vi "AlliGator Decay Window.vi"() -> ()   [LabVIEW 2021, in "AlliGator Local Decay Window.lvlib"]
doc: "Local Decay Window UI.\nThis window displays the decay (and when available, IRF, fit and residuals) at the selected ROI."
uses:
  AlliGator Local Decay Window.lvlib
  AlliGator Variables List.ctl
  AlliGator Local Decay Graph Window Event Refnum.ctl
  AlliGator Local Decay Fit Results.ctl
  AlliGator Image Profile Plot Data.ctl
  Graphs/XY Graph/XY Plot Data.ctl
  Graphs/XY Graph/XY Graph Refnum.ctl
  Graphs/XY Graph/XY Graph Event.ctl
  <vilib>/Utility/miscctls.llb/LVPoint32TypeDef.ctl
  Variant/Variant to Data/Variant to Boolean.vi
  Graphs/XY Graph/XY Graph Add-Ons.lvlib
  AlliGator Globals, Variables & Constants.lvlib
  AlliGator Image Profile Window.lvlib
  Notebook/Notebook.lvlib
  Rich Text Box/Rich Text Box.lvlib
  AlliGator Settings.lvlib
  Error/Error.lvlib
  Variant/Variant to Data/Variant to Data.lvlib
panel:
  out "Local Decay Graph TipStrip":string
  out "Local Decay Graph":cluster{"X Array":dbl[], "Y Array":dbl[]}[](graph)
  out "Expand top panel to increase Graph size/Expand lower panel to see fit results":string
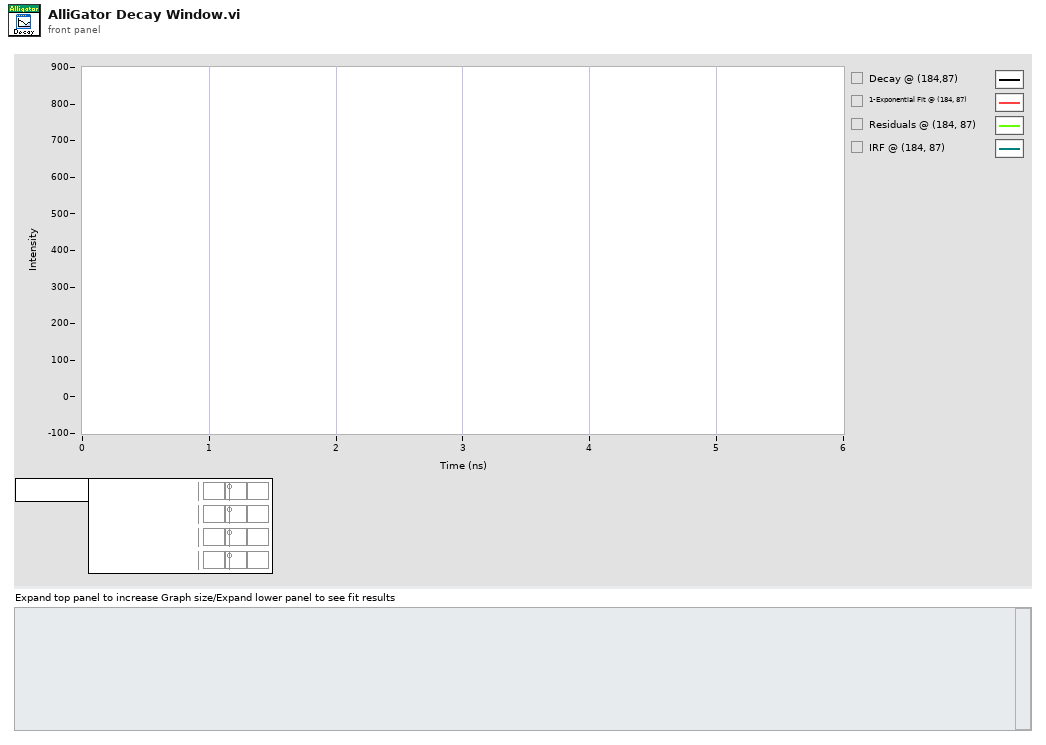
[diagram p1: front panel]
types:
  T1 = cluster{"Local Decay TipStrip Event":refnum<event-registration>, "Local Decay Window Event":refnum<event-registration>}
  T2 = typedef "AlliGator Local Decay Window.lvlib/AlliGator Local Decay Graph Window Event Refnum.ctl" = refnum<user-event>
  T3 = typedef "AlliGator Globals, Variables & Constants.lvlib/AlliGator Variables List.ctl" = enum16{"---- GUI ----", "Initialization Status", "State Indicators Refnum", "Original AlliGator Menu Items", "Current Action Loop State", "Script in progress", "Playback", "Loop Playback", "Search ROI Used", "Search ROI", "Decay Graph Max Legend Size", "Intensity Graph Max Legend Size", "Decay Statistics Graph Max Legend Size", "Phasor Graph Max Legend Size", "Phasor Ratio Graph Max Legend Size", "Lifetime Graph Max Legend Size", "---- Files ----", "Export Dataset Frames as Individual Files", "Show Batch Export Help Balloons", "Frames in Dataset", "ptu File Frame Start Indices", "Current Frame in Dataset", "Current Frame Timestamp", "------ Python Plugins ------", "Python Plugins Information", "Python Session", "Valid Python Session?", "---- Source Image ----", "Dataset Loaded", "Dataset Metadata", "Dataset Channel", "Dataset Data Description", "Background Dataset Metadata", "Background Dataset Channel", "Background Dataset Data Description", "Background File Subtraction", "Background File Path", "Background File Pile-up Correction", "Background File Pixel Well Capacity", "Background File Scaling Factor", "Source Image ROIs", "Current Source Image ROI", "Source Image ROI Event Refnum", "X_Source Image Display Range", "X_Source Image Palette Information", "Source Image Palette List", "Source Image Scale", "Current Dataset Load Settings", "Source Image:ROI Overlay Color", "---- Image Profile Window ----", "Image Profile:Overlay ROI in Source Image", "Image Profile Window Event Refnum", "Image Profile:IntensityType", "Image Profile:Intensity Average Type", "Image Profile:Intensity-weighted SDV", "Image Profile:Box Profile Type", "Image Profile Window Open", "Image Profile:Plotted Fit Parameter", "X_Type of Displayed Image", "X_Time Gate Slider", "Dataset Path", "Source Image Overlay to Erase", "Is Displayed Image Accumulated", "White Light Image Modified", "Mask Image Modified", "Macrotime Gate Separation", "------ Phasor Graph -------", "Phasor Graph:Show Line", "---- Phasor Plot ---", "Phasor Plot Parameters Changed", "FLI Dataset Modified since last Phasor Plot Calculation", "Phasor Harmonics Data", "Selected Phasor Harmonics", "Phasor Harmonic Manager Event Refnum", "Phasor Plot ROIs", "Current Phasor Plot ROI", "Phasor Plot ROI Event Refnum", "Phasor Plot Image Reference Points", "Phasor Plot Computed", "Phasor Plot Palette Information", "Phasor Plot Palette List", "Phasor Ratio Palette Information", "Phasor Ratio Palette List", "Phasor Image Scale", "Phasor Plot Image Overlay to Erase", "Phasor Plot Image Elements to Update", "Current Phasor Plot Calculation Parameters", "Current Phasor Calibration Options", "Reset Cumulated Phasor Plot", "Phasor Ratio Reference 1", "Phasor Ratio Lifetime Reference 1", "Phasor Ratio Reference 1 Frequency", "Phasor Ratio Reference 2", "Phasor Ratio Lifetime Reference 2", "Phasor Ratio Reference 2 Frequency", "---- Decay Analysis ----", "Number of Selected Decays to Fit", "LS Fit Results", "LAR Fit Results", "BS Fit Results", "Last Decay Max - Min", "Best Fit Parameters", "Best Fit Parameter Names", "Actual Size X", "Actual Size Y", "Binning X", "Binning Y", "Actual # Gates", "Dataset Number", "Gates to...", "Gates Skipped", "Gates to keep", "Gate Step", "Gate Separation", "Reversed Gates", "Pile-up Correction", "Pixel Well Capacity", "Background Subtracted", "Background Subtraction Method", "Background Definition Range", "Background File (deprecated)", "Number of Dataset Accumulated", "Array of Accumulated Dataset Paths", "Do Averaged Datasets", "Destination File Path", "Process Plot Target", "Use 1/D as Phasor Frequency", "---- Decay Fit Parameter Map -----", "Decay Fit Parameter Map Palette Information", "Decay Fit Parameter Map Palette List", "Local Decay Graph Window Event Refnum", "------- Local Decay Window ---------", "Use normalized IRF for convolution", "----- Miscellaneous ----", "Skippable Dialog Windows Status"}
  T4 = typedef "XY Graph Add-Ons.lvlib/XY Graph Refnum.ctl" = refnum<vi>
  T5 = typedef "XY Graph Add-Ons.lvlib/XY Graph Event.ctl" = cluster{"Item Tag":string, "XY Graph Refnum":refnum<vi>, "Coords":T6, "Item Path":string}
  T6 = typedef "LVPoint32TypeDef.ctl" = cluster{"Horizontal":i32, "Vertical":i32}
  T7 = typedef "Rich Text Box.lvlib/Text Formatting.ctl" = cluster{"Font":string, "Text Color":T8, "Text Background Color":T8, "Text Style":enum16{"Regular", "Bold", "Italic", "Underline", "Strikeout"}, "Font Size (Points)":dbl, "Text Alignment":i32}
  T8 = typedef "Rich Text Box.lvlib/Text Colors.ctl" = enum16{"Unchanged", "Black", "Blue", "Brown", "Gray", "Green", "Orange", "Pink", "Red", "White"}
  T9 = typedef "AlliGator Image Profile Window.lvlib/AlliGator Image Profile Plot Data.ctl" = cluster{"Plot Name":string, "Plot":T10}
  T10 = typedef "XY Graph Add-Ons.lvlib/XY Plot Data.ctl" = cluster{"X Array":dbl[], "Y Array":dbl[]}
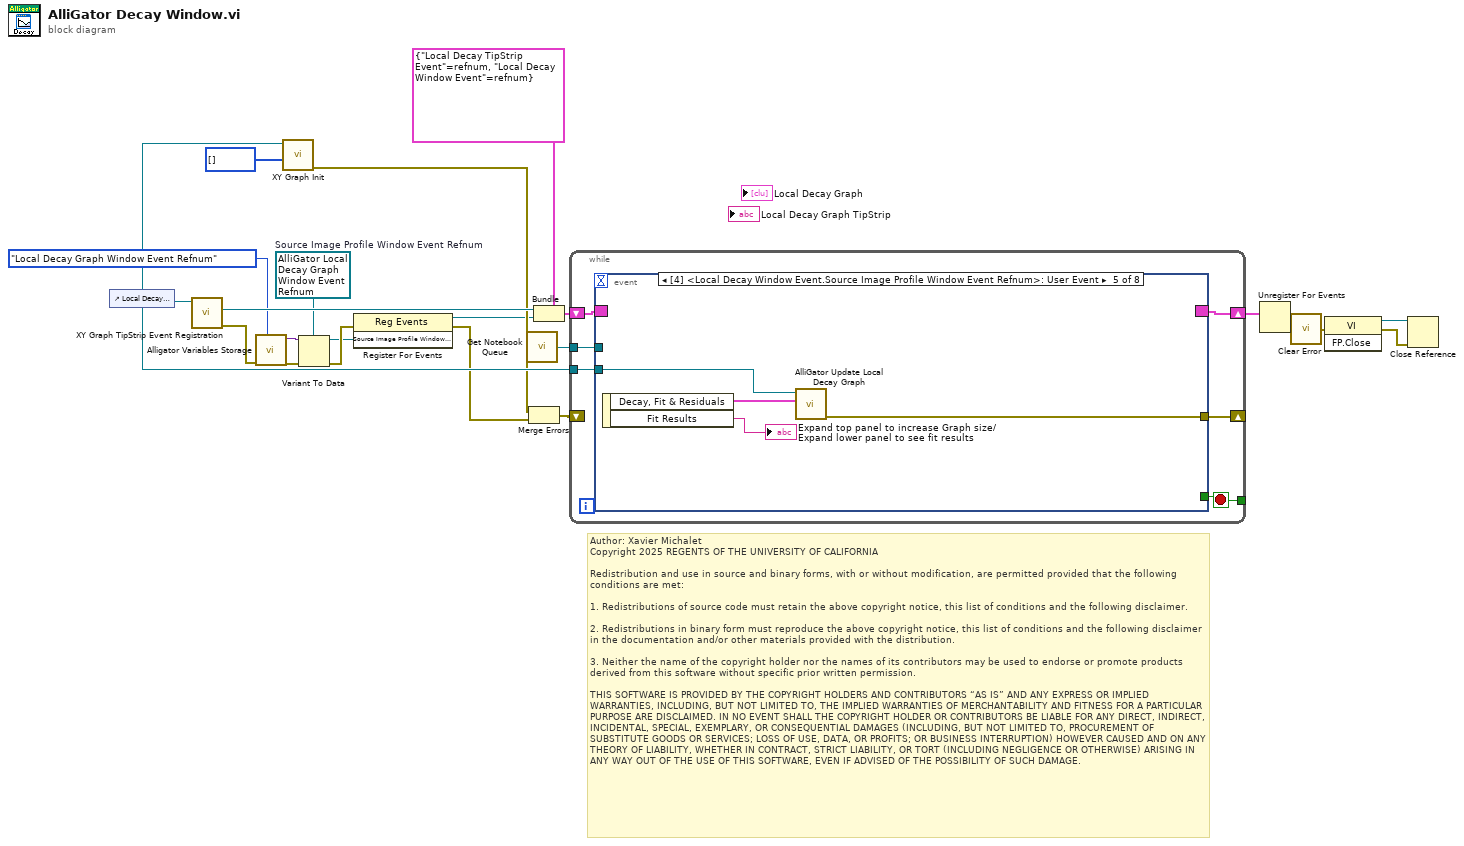
[diagram p0: block diagram]
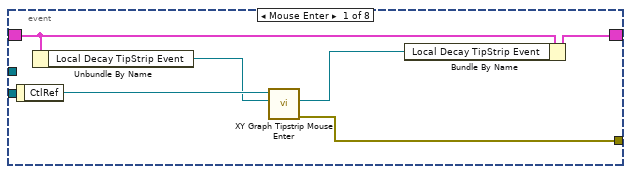
[diagram p2: hidden frame]
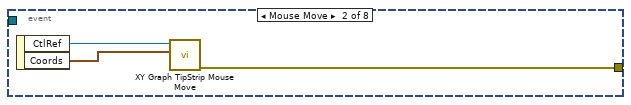
[diagram p3: hidden frame]
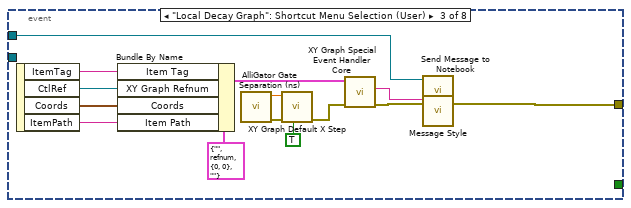
[diagram p4: hidden frame]
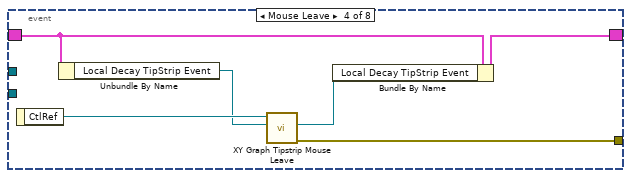
[diagram p5: hidden frame]
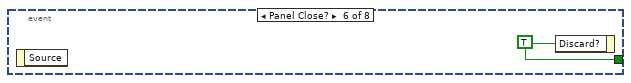
[diagram p6: hidden frame]
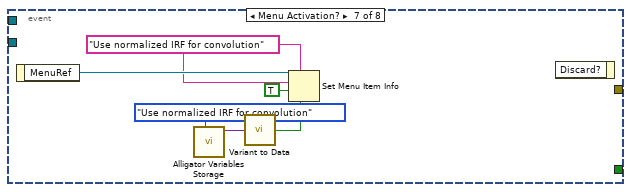
[diagram p7: hidden frame]
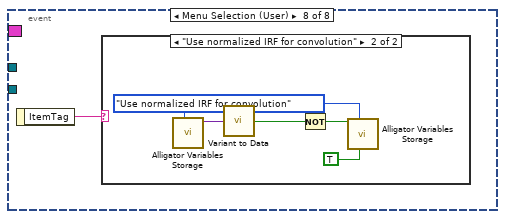
[diagram p8: hidden frame]
diagram:
  w15 = T2 refnum  # Source Image Profile Window Event Refnum
  # "Author: Xavier Michalet\nCopyright 2025 REGENTS OF THE UNIVERSITY OF CALIFORNIA\n\nRedistribution and use in source and binary forms, with or without modification, are permitted provided that the following conditions are met:\n\n1. Redistributions of source code must retain the above copyright notice, this list of conditions and the following disclaimer.\n\n2. Redistributions in binary form must reproduce the above copyright notice, this list of conditions and the following disclaimer in the documentation and/or other materials provided with the distribution.\n\n3. Neither the name of the copyright holder nor the names of its contributors may be used to endorse or promote products derived from this software without specific prior written permission.\n\nTHIS SOFTWARE IS PROVIDED BY THE COPYRIGHT HOLDERS AND CONTRIBUTORS “AS IS” AND ANY EXPRESS OR IMPLIED WARRANTIES, INCLUDING, BUT NOT LIMITED TO, THE IMPLIED WARRANTIES OF MERCHANTABILITY AND FITNESS FOR A PARTICULAR PURPOSE ARE DISCLAIMED. IN NO EVENT SHALL THE COPYRIGHT HOLDER OR CONTRIBUTORS BE LIABLE FOR ANY DIRECT, INDIRECT, INCIDENTAL, SPECIAL, EXEMPLARY, OR CONSEQUENTIAL DAMAGES (INCLUDING, BUT NOT LIMITED TO, PROCUREMENT OF SUBSTITUTE GOODS OR SERVICES; LOSS OF USE, DATA, OR PROFITS; OR BUSINESS INTERRUPTION) HOWEVER CAUSED AND ON ANY THEORY OF LIABILITY, WHETHER IN CONTRACT, STRICT LIABILITY, OR TORT (INCLUDING NEGLIGENCE OR OTHERWISE) ARISING IN ANY WAY OUT OF THE USE OF THIS SOFTWARE, EVEN IF ADVISED OF THE POSSIBILITY OF SUCH DAMAGE."
  n1 = control-ref of="Local Decay Graph"() -> (w19:refnum<vi>)
  n2 = call "XY Graph TipStrip Event Registration.vi"("XY Graph Refnum"=w19) -> ("error out"=w9:errorcluster, "Event Registration Refnum"=w21:refnum<event-registration>, "XY Graph Refnum"=w20:T4)  [unwired: 8 in]
  n3 = call "Alligator Variables Storage.vi"("AlliGator Variable"=AlliGator_Variables_List."Local Decay Graph Window Event Refnum" ("Alligator Variable"), "Error In"=w9) -> ("Error Out"=w16:errorcluster, "Data out"=w17:variant)  [unwired: 7 in, 1 out]
  n4 = call "XY Graph Init.vi"("Plots to Skip (none)"=i32[] [], "XYGraph in"=w20) -> ("Error Out"=w8:errorcluster)  [unwired: 9 in]
  n5 = Variant To Data(error in=w16, type=w15, Variant=w17) -> (data=w6:T2, error out=w14:errorcluster)
  n6 = register-events(error in=w14, w6) -> (reference out=w7:refnum<event-registration>, error out=w5:errorcluster)  [unwired: 1 in]
  n7 = call "Get Notebook Queue.vi"() -> ("Notebook Queue"=w11:refnum<queue>)  [unwired: 9 in]
  n8 = Merge Errors(w8, w5) -> (w10:errorcluster)
  n9 = Bundle(cluster=T1 {"Local Decay TipStrip Event"=refnum, "Local Decay Window Event"=refnum}, "Local Decay TipStrip Event"=w21, "Local Decay Window Event"=w7) -> (w12:T1)
  n10 = while {
    shift-right: [w28] -> w22
    shift-left: w12 -> [w29]
    tunnel: w19 -> [w27]
    tunnel: w11 -> [w26]
    shift-right: [w25] -> _
    shift-left: w10 -> [_]
    tunnel: [w24] -> _
    stop <- w24 stop-if-true
    n11 = event shown="[4] <Local Decay Window Event.Source Image Profile Window Event Refnum>: User Event" {
      selector: w29 -> [w33 _ _ w56 _ _ _ _]
      dyn-events: [w35 _ _ w55 _ _ _ _] -> w28
      timeout: _ -> [_ _ _ _ _ _ _ _]
      tunnel: [_ _ _ _ _ w64 _ _] -> w24
      tunnel: w27 -> [_ _ _ _ w63 _ _ _]
      tunnel: w26 -> [_ _ w51 _ _ _ _ _]
      tunnel: [w30 w36 w49 w54 w62 _ _ _] -> w25
      event Mouse Enter {
        n12 = event-data() -> ("CtlRef"=w34:refnum<vi>)  [unwired: 1 in]
        n13 = Unbundle By Name(w33) -> ("Local Decay TipStrip Event"=w32:refnum<event-registration>)
        n14 = call "XY Graph Tipstrip Mouse Enter.vi"("Event Registration Refnum"=w32, "XY Graph Refnum"=w34) -> ("Error Out"=w30:errorcluster, "Event Registration Refnum"=w31:refnum<event-registration>)  [unwired: 8 in]
        n15 = Bundle By Name(cluster=w33, "Local Decay TipStrip Event"=w31) -> (w35:T1)
      }
      event Mouse Move {
        n16 = event-data() -> ("CtlRef"=w38:refnum<vi>, "Coords"=w37:T6)  [unwired: 1 in]
        n17 = call "XY Graph TipStrip Mouse Move.vi"("Coords"=w37, "XY Graph Refnum"=w38) -> ("Error Out"=w36:errorcluster)  [unwired: 7 in, 2 out]
      }
      event "Local Decay Graph": Shortcut Menu Selection (User) {
        n18 = event-data() -> ("ItemTag"=w48:string, "CtlRef"=w47:refnum<vi>, "Coords"=w46:T6, "ItemPath"=w45:string)  [unwired: 1 in]
        n19 = Bundle By Name(cluster=T5 {"Item Tag"="", "XY Graph Refnum"=refnum, "Coords"={"Horizontal"=0, "Vertical"=0}, "Item Path"=""} ("XY Graph Event"), "Item Tag"=w48, "XY Graph Refnum"=w47, "Coords"=w46, "Item Path"=w45) -> (w43:T5)
        n20 = call "AlliGator Gate Separation (ns).vi"() -> ("error out"=w42:errorcluster, "Gate Separation (ns)"=w40:dbl)  [unwired: 10 in]
        n21 = call "XY Graph Default X Step.vi"("Get (F)/Set"=TRUE, "Error In"=w42, "Default X Step"=w40) -> ("Error Out"=w41:errorcluster)  [unwired: 7 in, 1 out]
        n22 = call "XY Graph Special Event Handler Core.vi"("error in (no error)"=w41, "XY Graph Event"=w43) -> ("error out"=w53:errorcluster, "Message"=w52:string)  [unwired: 5 in, 3 out]
        n23 = call "Message Style.vi"() -> ("Message Formatting"=w50:T7)
        n24 = call "Send Message to Notebook.vi"("Text Formatting"=w50, "Error In"=w53, "Message"=w52, "Notebook Queue"=w51) -> ("Error Out"=w49:errorcluster)  [unwired: 4 in, 1 out]
      }
      event Mouse Leave {
        n25 = event-data() -> ("CtlRef"=w59:refnum<vi>)  [unwired: 1 in]
        n26 = Unbundle By Name(w56) -> ("Local Decay TipStrip Event"=w58:refnum<event-registration>)
        n27 = call "XY Graph Tipstrip Mouse Leave.vi"("Event Registration Refnum"=w58, "XY Graph Refnum"=w59) -> ("Error Out"=w54:errorcluster, "Event Registration Refnum"=w57:refnum<event-registration>)  [unwired: 8 in]
        n28 = Bundle By Name(cluster=w56, "Local Decay TipStrip Event"=w57) -> (w55:T1)
      }
      event User Event {
        n29 = event-data() -> ("Decay, Fit & Residuals"=w61:T9[], "Fit Results"=→"Expand top panel to increase Graph size/Expand lower panel to see fit results":string)  [unwired: 1 in]
        n30 = call "AlliGator Update Local Decay Graph.vi"("Profile Window Data"=w61, "XY Graph Refnum"=w63) -> ("Error Out"=w62:errorcluster)  [unwired: 9 in]
      }
      event Panel Close? {
        w64 = TRUE ("Discard?")
        n31 = event-data() -> ()  [unwired: 1 in, 1 out]
        n32 = event-data("Discard?"=w64) -> ()  [unwired: 1 in, 1 out]
      }
      event Menu Activation? {
        w66 = "Use normalized IRF for convolution" ("item tag")
        n33 = event-data() -> ("MenuRef"=w70:refnum<k9>)  [unwired: 1 in]
        n34 = call "Alligator Variables Storage.vi"("AlliGator Variable"=AlliGator_Variables_List."Use normalized IRF for convolution") -> ("Data out"=w68:variant)  [unwired: 8 in, 2 out]
        n35 = call-poly "Variant to Data.vi"("Variant"=w68) -> ("Value"=w67:bool)  [unwired: 8 in]
        n36 = Set Menu Item Info(6:w67, 7:w66, 9:TRUE ("enabled"), 10:w66, 11:w70) -> ()  [unwired: 2 in, 2 out]
        n37 = event-data() -> ()  [unwired: 2 in, 1 out]
      }
      event Menu Selection (User) {
        n38 = event-data() -> ("ItemTag"=w71:string)  [unwired: 1 in]
        n39 = case shown="\"Use normalized IRF for convolution\"" w71 {
          frame "", Default {
          }
          frame "Use normalized IRF for convolution" {
            w72 = AlliGator_Variables_List."Use normalized IRF for convolution" ("AlliGator Variable")
            n40 = call "Alligator Variables Storage.vi"("AlliGator Variable"=w72) -> ("Data out"=w76:variant)  [unwired: 8 in, 2 out]
            n41 = call-poly "Variant to Data.vi"("Variant"=w76) -> ("Value"=w75:bool)  [unwired: 8 in]
            n42 = Not(x=w75) -> (.not. x?=w74:bool)
            n43 = call "Alligator Variables Storage.vi"("Get(F)/Set"=TRUE, "AlliGator Variable"=w72, "Data in"=w74) -> ()  [unwired: 6 in, 3 out]
          }
        }
      }
    }
  }
  n44 = Unregister For Events(event registration refnum=w22) -> (error out=w4:errorcluster)  [unwired: 1 in]
  n45 = call "Clear Error.vi"("Error In"=w4) -> ("no Error Out"=w1:errorcluster)  [unwired: 8 in]
  n46 = invoke class="VI" method="FP.Close"(error in=w1) -> (reference out=w2:refnum<vi>, error out=w3:errorcluster)  [unwired: 2 in, 1 out]
  n47 = Close Reference(reference=w2, error in (no error)=w3) -> ()  [unwired: 1 out]
